vi "Configure Modulation (Phase).vi"(4 "Peak Deviation (180 Degrees)":i32=180 min=0 max=180, 6 "Modulation Frequency (10 Hz)":dbl=10.0, 7 "Enable Pulse Modulation (T:Enable)":bool=TRUE, 8 "error in (no error)":errorcluster, 9 "Modulation Waveform (Sine)":T1(ring), 10 "PM Source (Internal)":enum16{"Internal", "External"}(ring), 11 "VISA resource name":refnum<visa-resource-name>) -> (0 "error out":errorcluster, 3 "VISA resource name out":refnum<visa-resource-name>)   [LabVIEW 2017, in "Keithley 3390.lvlib"]
doc: "Configures and enables phase modulation (PM). In PM, the phase of the carrier is varied by the frequency of the modulating waveform. \n\n<B>Note:</B> The carrier waveform shape and parameters are set by the Configure Waveform VI."
uses:
  Keithley 3390.lvlib
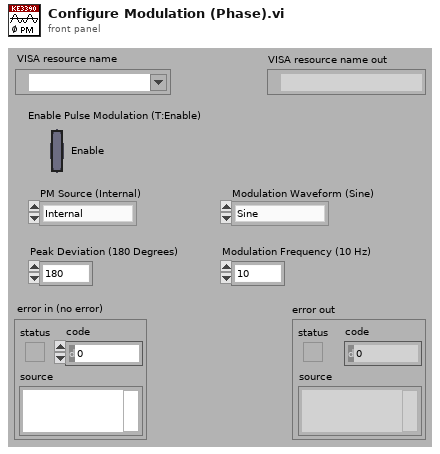
[diagram p1: front panel]
types:
  T1 = enum16{"Sine", "Square", "Ramp", "Negative Ramp", "Triangle", "Noise", "Arbitrary"}
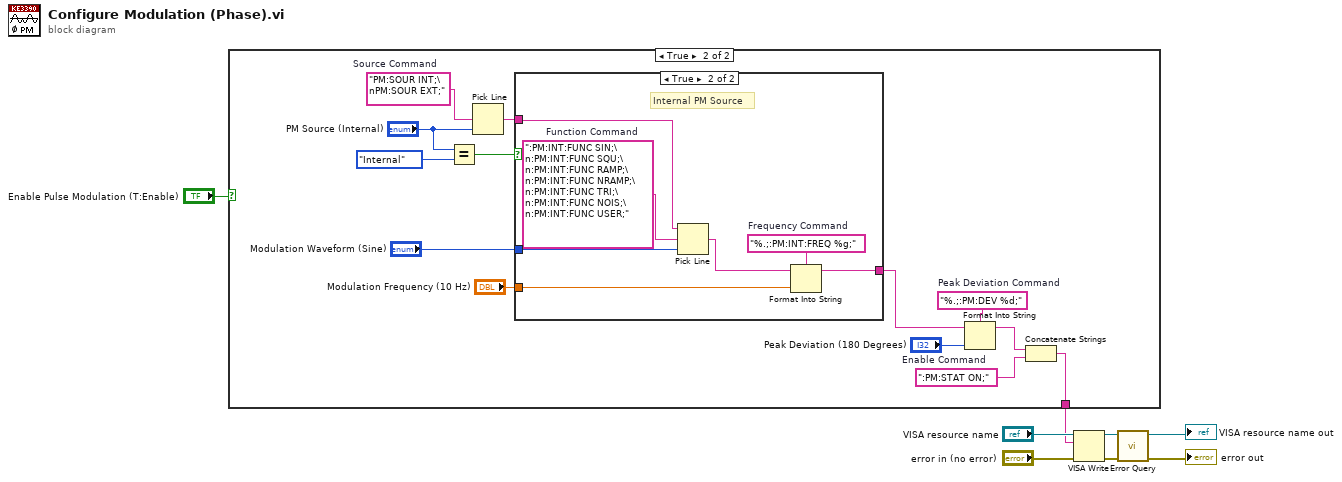
[diagram p0: block diagram]
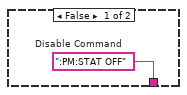
[diagram p2: hidden frame]
diagram:
  n1 = case shown="True" "Enable Pulse Modulation (T:Enable)" {
    tunnel: [w9 w13] -> w6
    frame False {
      w9 = ":PM:STAT OFF"  # Disable Command
    }
    frame True {
      w11 = ":PM:STAT ON;"  # Enable Command
      w18 = "PM:SOUR INT;\nPM:SOUR EXT;"  # Source Command
      w21 = "%.;:PM:DEV %d;"  # Peak Deviation Command
      n2 = Equal?(x="PM Source (Internal)", y=enum16{"Internal", "External"}."Internal") -> (x = y?=w16:bool)
      n3 = Pick Line(multi-line string=w18, line index="PM Source (Internal)") -> (output string=w15:string)  [unwired: 1 in]
      n4 = case shown="True" w16 {
        tunnel: [w23 w28] -> w20
        tunnel: "Modulation Frequency (10 Hz)" -> [_ w27]
        tunnel: w15 -> [w23 w25]
        tunnel: "Modulation Waveform (Sine)" -> [_ w24]
        frame False {
          # "External PM Source"
        }
        frame True {
          w26 = ":PM:INT:FUNC SIN;\n:PM:INT:FUNC SQU;\n:PM:INT:FUNC RAMP;\n:PM:INT:FUNC NRAMP;\n:PM:INT:FUNC TRI;\n:PM:INT:FUNC NOIS;\n:PM:INT:FUNC USER;"  # Function Command
          w30 = "%.;:PM:INT:FREQ %g;"  # Frequency Command
          # "Internal PM Source"
          n5 = Pick Line(string ("")=w25, multi-line string=w26, line index=w24) -> (output string=w29:string)
          n6 = Format Into String(format string=w30, initial string=w29, w27) -> (resulting string=w28:string)  [unwired: 1 in, 1 out]
        }
      }
      n7 = Format Into String(format string=w21, initial string=w20, "Peak Deviation (180 Degrees)") -> (resulting string=w12:string)  [unwired: 1 in, 1 out]
      n8 = Concatenate Strings(w12, w11) -> (w13:string)
    }
  }
  n9 = VISA Write(VISA resource name="VISA resource name", write buffer=w6, error in (no error)="error in (no error)") -> (VISA resource name out=w4:refnum<visa-resource-name>, error out=w5:errorcluster)  [unwired: 1 out]
  n10 = call "Error Query.vi"("error in (no error)"=w5, "VISA resource name"=w4) -> ("error out"=→"error out":errorcluster, "VISA resource name out"=→"VISA resource name out":refnum<visa-resource-name>)  [unwired: 6 in, 2 out]
